vi "Class Write.vi"(4 "error in (no error)":errorcluster, 5 "Value":refnum<class "MGI Path Selector.lvclass">, 6 "Container State":T2, 7 "Display State In":T1) -> (0 "error out":errorcluster, 3 "Display State Out":T1)   [LabVIEW 2016, in "MGI Path Selector.xctl"]
uses:
  <userlib>/_MGI/User Interface/Path Selector XControl/MGI Path Selector.xctl
  <vilib>/_xctls/Container State.ctl
  <userlib>/_MGI/User Interface/Path Selector XControl/Class Hierarchy/MGI Path Selector.lvclass
  <userlib>/_MGI/User Interface/Path Selector XControl/State.ctl
  <vilib>/_xctls/XControlSupport.lvlib
panel:
  # "Replace the Value Control below with a Control of desired type.\nDo not remove this Control or the others from the connector pane.\nDo not change the connector pane pattern.\nThe Value control should always be the third terminal from top on the input side in the connector pane."
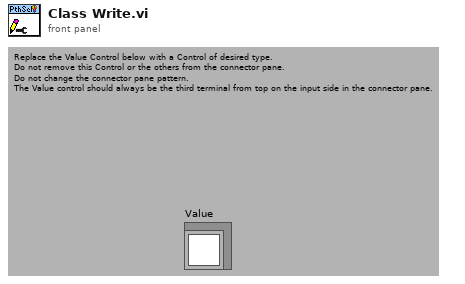
[diagram p1: front panel]
types:
  T1 = typedef "MGI Path Selector.xctl/State.ctl" = cluster{"Class":refnum<class "MGI Path Selector.lvclass">, "Persist":string}
  T2 = typedef "XControlSupport.lvlib/Container State.ctl" = cluster{"Indicator?":bool, "Run Mode?":bool, " Refnum":refnum<vi>}
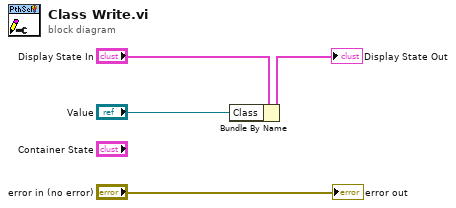
[diagram p0: block diagram]
diagram:
  n1 = Bundle By Name(cluster="Display State In", "Class"="Value") -> (→"Display State Out":T1)
  "error out" <- "error in (no error)"
